vi "Read property By Key.vi"(10 "key":string, 11 "TestManagerMsg.Test in":refnum<class "TestManagerMsg.Test.lvclass">) -> (1 "found":bool, 2 "property":refnum<class "TestManagerMsg.KVP.lvclass">, 3 "TestManagerMsg.Test out":refnum<class "TestManagerMsg.Test.lvclass">)   [LabVIEW 2020, in "Caraya.lvlib" / "TestManagerMsg.Test.lvclass"]
uses:
  TestManagerMsg.Test.lvclass
  Test Manager Message KVP/TestManagerMsg.KVP.lvclass
  TestManagerMsg.Test.lvclass/TestManagerMsg.Test.ctl
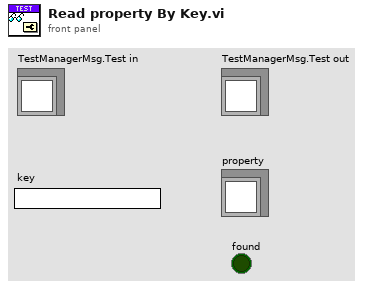
[diagram p1: front panel]
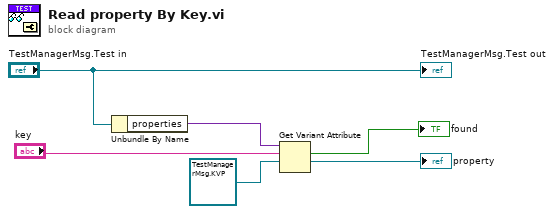
[diagram p0: block diagram]
diagram:
  n1 = Unbundle By Name("TestManagerMsg.Test in") -> ("properties"=w5:variant)
  n2 = Get Variant Attribute(Variant=w5, name="key", default value (empty Variant)=refnum<class "TestManagerMsg.KVP.lvclass"> refnum ("KVP")) -> (found=→"found":bool, value=→"property":refnum<class "TestManagerMsg.KVP.lvclass">)  [unwired: 1 in, 2 out]
  "TestManagerMsg.Test out" <- "TestManagerMsg.Test in"
